vi "Stimulus-Create (array).vi"(0 "AO Control":T1[](xcontrol), 1 "Apply multipliers? (F)":bool, 5 "Sampling Rate (Hz)":dbl=100000.0, 7 "Npts":i32=500, 11 "error in (no error)":errorcluster) -> (4 "AO Control out":T1[](xcontrol), 6 "Waveform":dbl[][](array[numeric]), 15 "error out":errorcluster)   [LabVIEW 2015]
uses:
  Controls/Multichannel XCtl/Multichannel XCtl.xctl
  PXI DAQ VIs/DAQ Engine VIs/AO Gain and Multiplier VIs/PXI Multipliers to AO Gains (1D).vi
panel:
  out "Ceilings":dbl[](array[numeric])
  out "Gains":dbl[](array[numeric])
  out "Multipliers":dbl[](array[numeric])
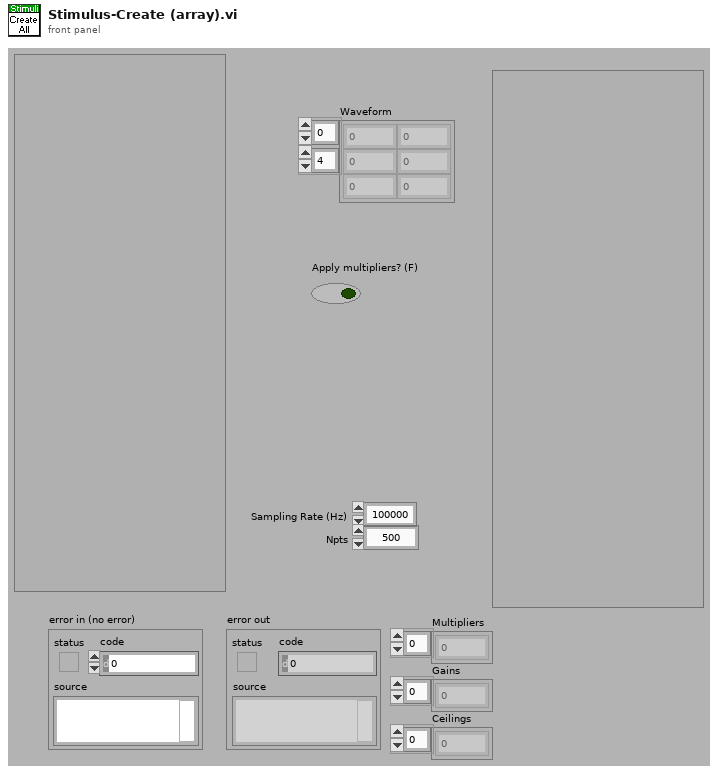
[diagram p1: front panel]
types:
  T1 = typedef "Stimulus Channel.xctl/Stimulus Channel Data.ctl" = cluster{"Waveform":T2, "Filter":T16, "Gate":T17, "Level":T18}
  T2 = typedef "Waveform XCtl.xctl/Waveform Data.ctl" = cluster{"Type":T3, "Tone":T4, "Pulse Train":T5, "Noise":T8, "File":T9, "FMSweep":T10, "Chirp Train":T11, "Complex Tone":cluster{"Params":T13, "Data":T15}}
  T3 = typedef "Waveform Enum.ctl" = enum16{"OFF", "Tone", "Noise", "Pulse Train", "File", "FM Sweep", "Chirp Train", "Complex Tone"}
  T4 = typedef "Tone Params.ctl" = cluster{"Frequency (kHz)":dbl, "Last Freq":dbl, "Last Phase":dbl}
  T5 = typedef "Pulse Train Params.ctl" = cluster{"Pulse width (us)":dbl, "Pulse rate (Hz)":dbl, "Gap (ms)":dbl, "Polarity":T6, "PT State":T7, "Asynch":bool}
  T6 = typedef "Pulse Polarity.ctl" = enum16{"POS", "NEG", "POS-NEG", "NEG-POS"}
  T7 = typedef "PT-Continuous State.ctl" = cluster{"Template":dbl[], "Nperiod":i32, "Index":i32, "Pulse Rate (Hz)":dbl, "Phase (cycles)":dbl, "Noff":i32}
  T8 = typedef "Noise Params.ctl" = cluster{"InvFilt":bool, "Noise":dbl[], "CurPt":i32, "Aweight":bool}
  T9 = typedef "StimFile-Params.ctl" = cluster{"Filename":path, "Signal":dbl[], "Channel":i32}
  T10 = typedef "FM Sweep Params.ctl" = cluster{"Rate (oct/s)":dbl, "Fmin (Hz)":dbl, "Fmax (Hz)":dbl, "Ramp (ms)":dbl, "Linear":bool}
  T11 = typedef "Chirp Train.ctl" = cluster{"Params":T12, "Data":cluster{"WF":dbl[]}}
  T12 = typedef "Chirp Train Params.ctl" = cluster{"Fmin (kHz)":dbl, "Fmax (kHz)":dbl, "Compensate":bool, "Duration (ms)":dbl}
  T13 = typedef "CT-Params.ctl" = cluster{"F0 (Hz)":dbl, "Band":cluster{"Flow (Hz)":dbl, "Fhigh (Hz)":dbl}, "Phase":T14, "Min F0 (Hz)":dbl, "Max F0 (Hz)":dbl, "ContinRandPhase":bool, "Max peak factor":dbl, "Max mod depth":dbl}
  T14 = typedef "CT-Phase Enum.ctl" = enum16{"Cosine", "Random", "Alternating"}
  T15 = typedef "CT-Runtime Data.ctl" = cluster{"Ncomp":i32, "MinHarm":i32, "Phase":dbl[], "Amplitude":dbl[], "Npts/frame":i32, "Last F0":dbl, "Fmin":dbl, "Fmax":dbl, "Lslope":dbl, "randphase":bool}
  T16 = typedef "Filter XCtl.xctl/Filter Data.ctl" = cluster{"CF (kHz)":dbl, "BW (kHz)":dbl, "IIR Filter Cluster":cluster{"filter structure":enum32{"IIR 2nd Order", "IIR 4th Order"}, "Reverse Coefficients":dbl[], "Forward Coefficients":dbl[]}, "Final Filter State":dbl[], "Scale Factor":dbl, "Final Filter State 2":dbl[], "Quadrature":bool, "Type":enum16{"Lowpass", "Highpass", "Bandpass", "Bandstop", "OFF"}}
  T17 = typedef "Gate Control.xctl/Gate Data.ctl" = cluster{"Active":bool, "Delay (ms)":dbl, "Width (ms)":dbl, "Ramp (ms)":dbl}
  T18 = typedef "Level XCtl.xctl/Level Data.ctl" = cluster{"Level":dbl, "Units":T19, "Max":dbl, "Multiplier":dbl, "Cal File":path, "Cal":cluster{"Freq (Hz)":dbl[], "Mag (dB SPL)":dbl[], "Phase (deg)":dbl[]}}
  T19 = typedef "Level Units.ctl" = enum16{"dB atten", "dB SPL", "dB re 1 Vrms", "dB V/Hz½", "mW", "dB SL"}
  T20 = cluster{"Waveform":T2, "Filter":T16, "Gate":T17, "Level":T18}
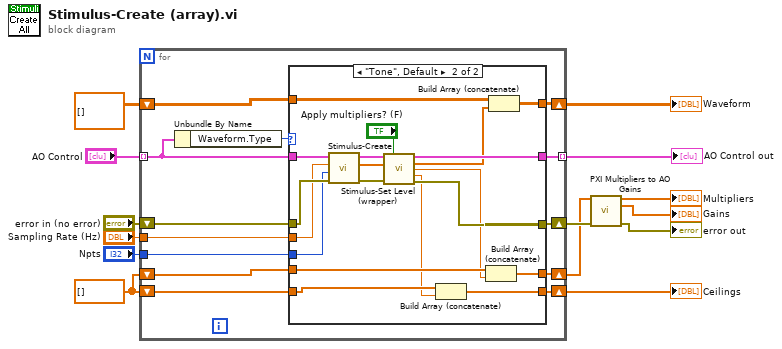
[diagram p0: block diagram]
diagram:
  w7 = dbl[] []
  n1 = for {
    tunnel: [w25] -> w4 mode=indexing
    shift-right: [w23] -> w1
    shift-left: dbl[][] [] ("Waveform") -> [w24]
    shift-right: [w21] -> w8
    shift-left: w7 -> [w22]
    shift-right: [w26] -> w13
    shift-left: "error in (no error)" -> [w27]
    shift-right: [w19] -> w6
    shift-left: w7 -> [w20]
    tunnel: "AO Control" -> [w18] mode=indexing
    tunnel: "Sampling Rate (Hz)" -> [w17]
    tunnel: "Npts" -> [w16]
    n2 = Unbundle By Name(w18) -> ("Waveform.Type"=w15:T3)
    n3 = case shown="\"Tone\", Default" w15 {
      tunnel: w27 -> [w31 w51]
      tunnel: [w31 w42] -> w26
      tunnel: [w28 w41] -> w25
      tunnel: w24 -> [w32 w49]
      tunnel: [w32 w50] -> w23
      tunnel: w22 -> [w30 w47]
      tunnel: [w30 w48] -> w21
      tunnel: w20 -> [w29 w45]
      tunnel: [w29 w46] -> w19
      tunnel: w18 -> [w28 w33]
      tunnel: w17 -> [_ w43]
      tunnel: w16 -> [_ w44]
      frame "OFF" {
      }
      frame "Tone", Default {
        n4 = call "Stimulus-Create.vi"("error in (no error)"=w51, "Npts"=w44, "Sampling Rate (Hz)"=w43, "Stimulus Channel"=w33) -> ("error out"=w39:errorcluster, "Waveform"=w38:dbl[], "Stimulus Channel out"=w40:T20)  [unwired: 4 in, 1 out]
        n5 = call "Stimulus-Set Level (wrapper).vi"("Stimulus Channel"=w40, "Apply multiplier? (F)"="Apply multipliers? (F)", "Waveform in"=w38, "error in (no error)"=w39) -> ("Stimulus Channel out"=w41:T20, "Waveform out"=w34:dbl[], "Multiplier"=w36:dbl, "Ceiling"=w37:dbl, "error out"=w42:errorcluster)  [unwired: 7 in]
        n6 = Build Array (concatenate)(w45, w37) -> (w46:dbl[])
        n7 = Build Array (concatenate)(w47, w36) -> (w48:dbl[])
        n8 = Build Array (concatenate)(w49, w34) -> (w50:dbl[][])
      }
    }
  }
  "Waveform" <- w1
  "AO Control out" <- w4
  "Ceilings" <- w6
  n9 = call-poly "PXI Multipliers to AO Gains.vi"("Multipliers in"=w8, "error in (no error)"=w13) -> ("Multipliers out"=→"Multipliers":dbl[], "Gains"=→"Gains":dbl[], "error out"=→"error out":errorcluster)  [unwired: 11 in]
